vi "emi_Check-Create Folders in path.vi"(0 "Path including file":path, 11 "error in (no error)":errorcluster) -> (4 "Path out":path, 8 "Folder tried created":bool, 15 "error out":errorcluster)   [LabVIEW 2011]
doc: "Provide a path, and the VI will create all nececery folders in it. Used in cases where a folder needs to be created, but one can not garenty that a parent folder exists.\n\nPath must include a file! The file will not be created.\nTo create E:/tull/tull/: Using path: E:/tull/tull/ wil only create E:/tull. Use : \"E:/tull/tull/dummy.any\" or something like that.\n\nIf a folder in the path can not be created, an error will be returned.\n\nOn error in: No folder will be created."
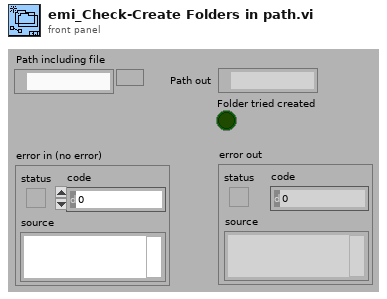
[diagram p1: front panel]
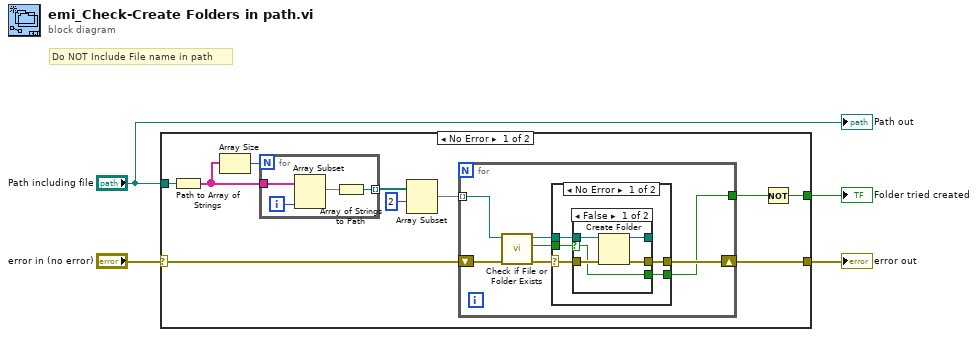
[diagram p0: block diagram]
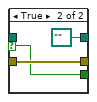
[diagram p2: hidden frame]
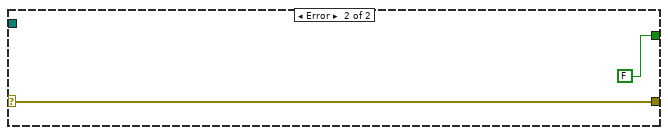
[diagram p4: hidden frame]
diagram:
  # "Do NOT Include File name in path"
  n1 = case shown="No Error" "error in (no error)" {
    selector: "error in (no error)" -> [w5 w41]
    tunnel: [w9 w41] -> w4
    tunnel: "Path including file" -> [w8 _]
    tunnel: [w6 FALSE] -> w2
    frame No Error {
      n2 = Path to Array of Strings(0:w8) -> (2:w13:string[])  [unwired: 1 out]
      n3 = Array Size(array=w13) -> (size(s)=w14:i32)
      n4 = for {
        N: w14 -> [_]
        tunnel: w13 -> [w40]
        tunnel: [w37] -> w12 mode=indexing
        i -> [w39]
        n5 = Array Subset(array=w40, length=w39) -> (w38:string[])  [unwired: 1 in]
        n6 = Array of Strings to Path(0:w38) -> (2:w37:path)  [unwired: 1 in]
      }
      n7 = Array Subset(array=w12, index=2) -> (w10:path[])  [unwired: 1 in]
      n8 = for {
        tunnel: w10 -> [w21] mode=indexing
        shift-right: [w17] -> w9
        shift-left: w5 -> [w20]
        tunnel: [w16] -> w7
        n9 = call <vilib>:"Check if File or Folder Exists.vi"("error in (no error)"=w20, "path"=w21) -> ("error out"=w15:errorcluster, "file or folder exists?"=w19:bool, "dup path"=w18:path)  [unwired: 7 in]
        n10 = case shown="No Error" w15 {
          selector: w15 -> [w22 w36]
          tunnel: w19 -> [w26 w35]
          tunnel: w18 -> [w25 _]
          tunnel: [w24 w36] -> w17
          tunnel: [w23 w35] -> w16
          frame No Error {
            n11 = case shown="False" w26 {
              selector: w26 -> [w28 w33]
              tunnel: w25 -> [w31 _]
              tunnel: w22 -> [w30 w34]
              tunnel: [w29 w34] -> w24
              tunnel: [w28 w33] -> w23
              tunnel: [w27 path "" ("created path")] -> _
              frame False {
                n12 = Create Folder(path (use dialog)=w31, error in=w30) -> (created path=w27:path, error out=w29:errorcluster)  [unwired: 1 in, 1 out]
              }
              frame True {
              }
            }
          }
          frame Error {
          }
        }
      }
      n13 = Not(x=w7) -> (.not. x?=w6:bool)
    }
    frame Error {
    }
  }
  "error out" <- w4
  "Folder tried created" <- w2
  "Path out" <- "Path including file"
